vi "UpdateLaserAOTFSettings.vi"(0 "3.LaserChannel ON/OFF":bool, 1 "4.LaserChannel ON/OFF":bool, 2 "On/OFF  Power 2":bool, 3 "6.LaserChannel ON/OFF":bool, 4 "7.LaserChannel ON/OFF":bool, 5 "8.LaserChannel ON/OFF":bool, 6 "1.Laser Channel Power / [%]":i16 min=0 max=100 step=1, 7 "2.Laser Channel Power / [%]":i16 min=0 max=100 step=1, 8 "2.LaserChannel ON/OFF":bool, 9 "3.Laser Channel Power / [%]":i16 min=0 max=100 step=1, 10 "On/OFF  Power":bool, 11 "4.Laser Channel Power / [%]":i16 min=0 max=100 step=1, 13 "5.Laser Channel Power / [%]":i16 min=0 max=100 step=1, 14 "error in":errorcluster, 15 "6.Laser Channel Power / [%]":i16 min=0 max=100 step=1, 17 "7.Laser Channel Power / [%]":i16 min=0 max=100 step=1, 19 "8.Laser Channel Power / [%]":i16 min=0 max=100 step=1, 20 "1.Laser Channel Wavelength 8":i32, 21 "1.Laser Channel Wavelength 7":i32, 22 "1.Laser Channel Wavelength 6":i32, 23 "Wavelength 2":i32, 24 "1.Laser Channel Wavelength 4":i32, 25 "1.Laser Channel Wavelength 3":i32, 26 "1.Laser Channel Wavelength 2":i32, 27 "Wavelength":i32) -> (18 "error out":errorcluster)   [LabVIEW 2013]
uses:
  Variables/AOTF_NonLinearLinesOnOff.vi
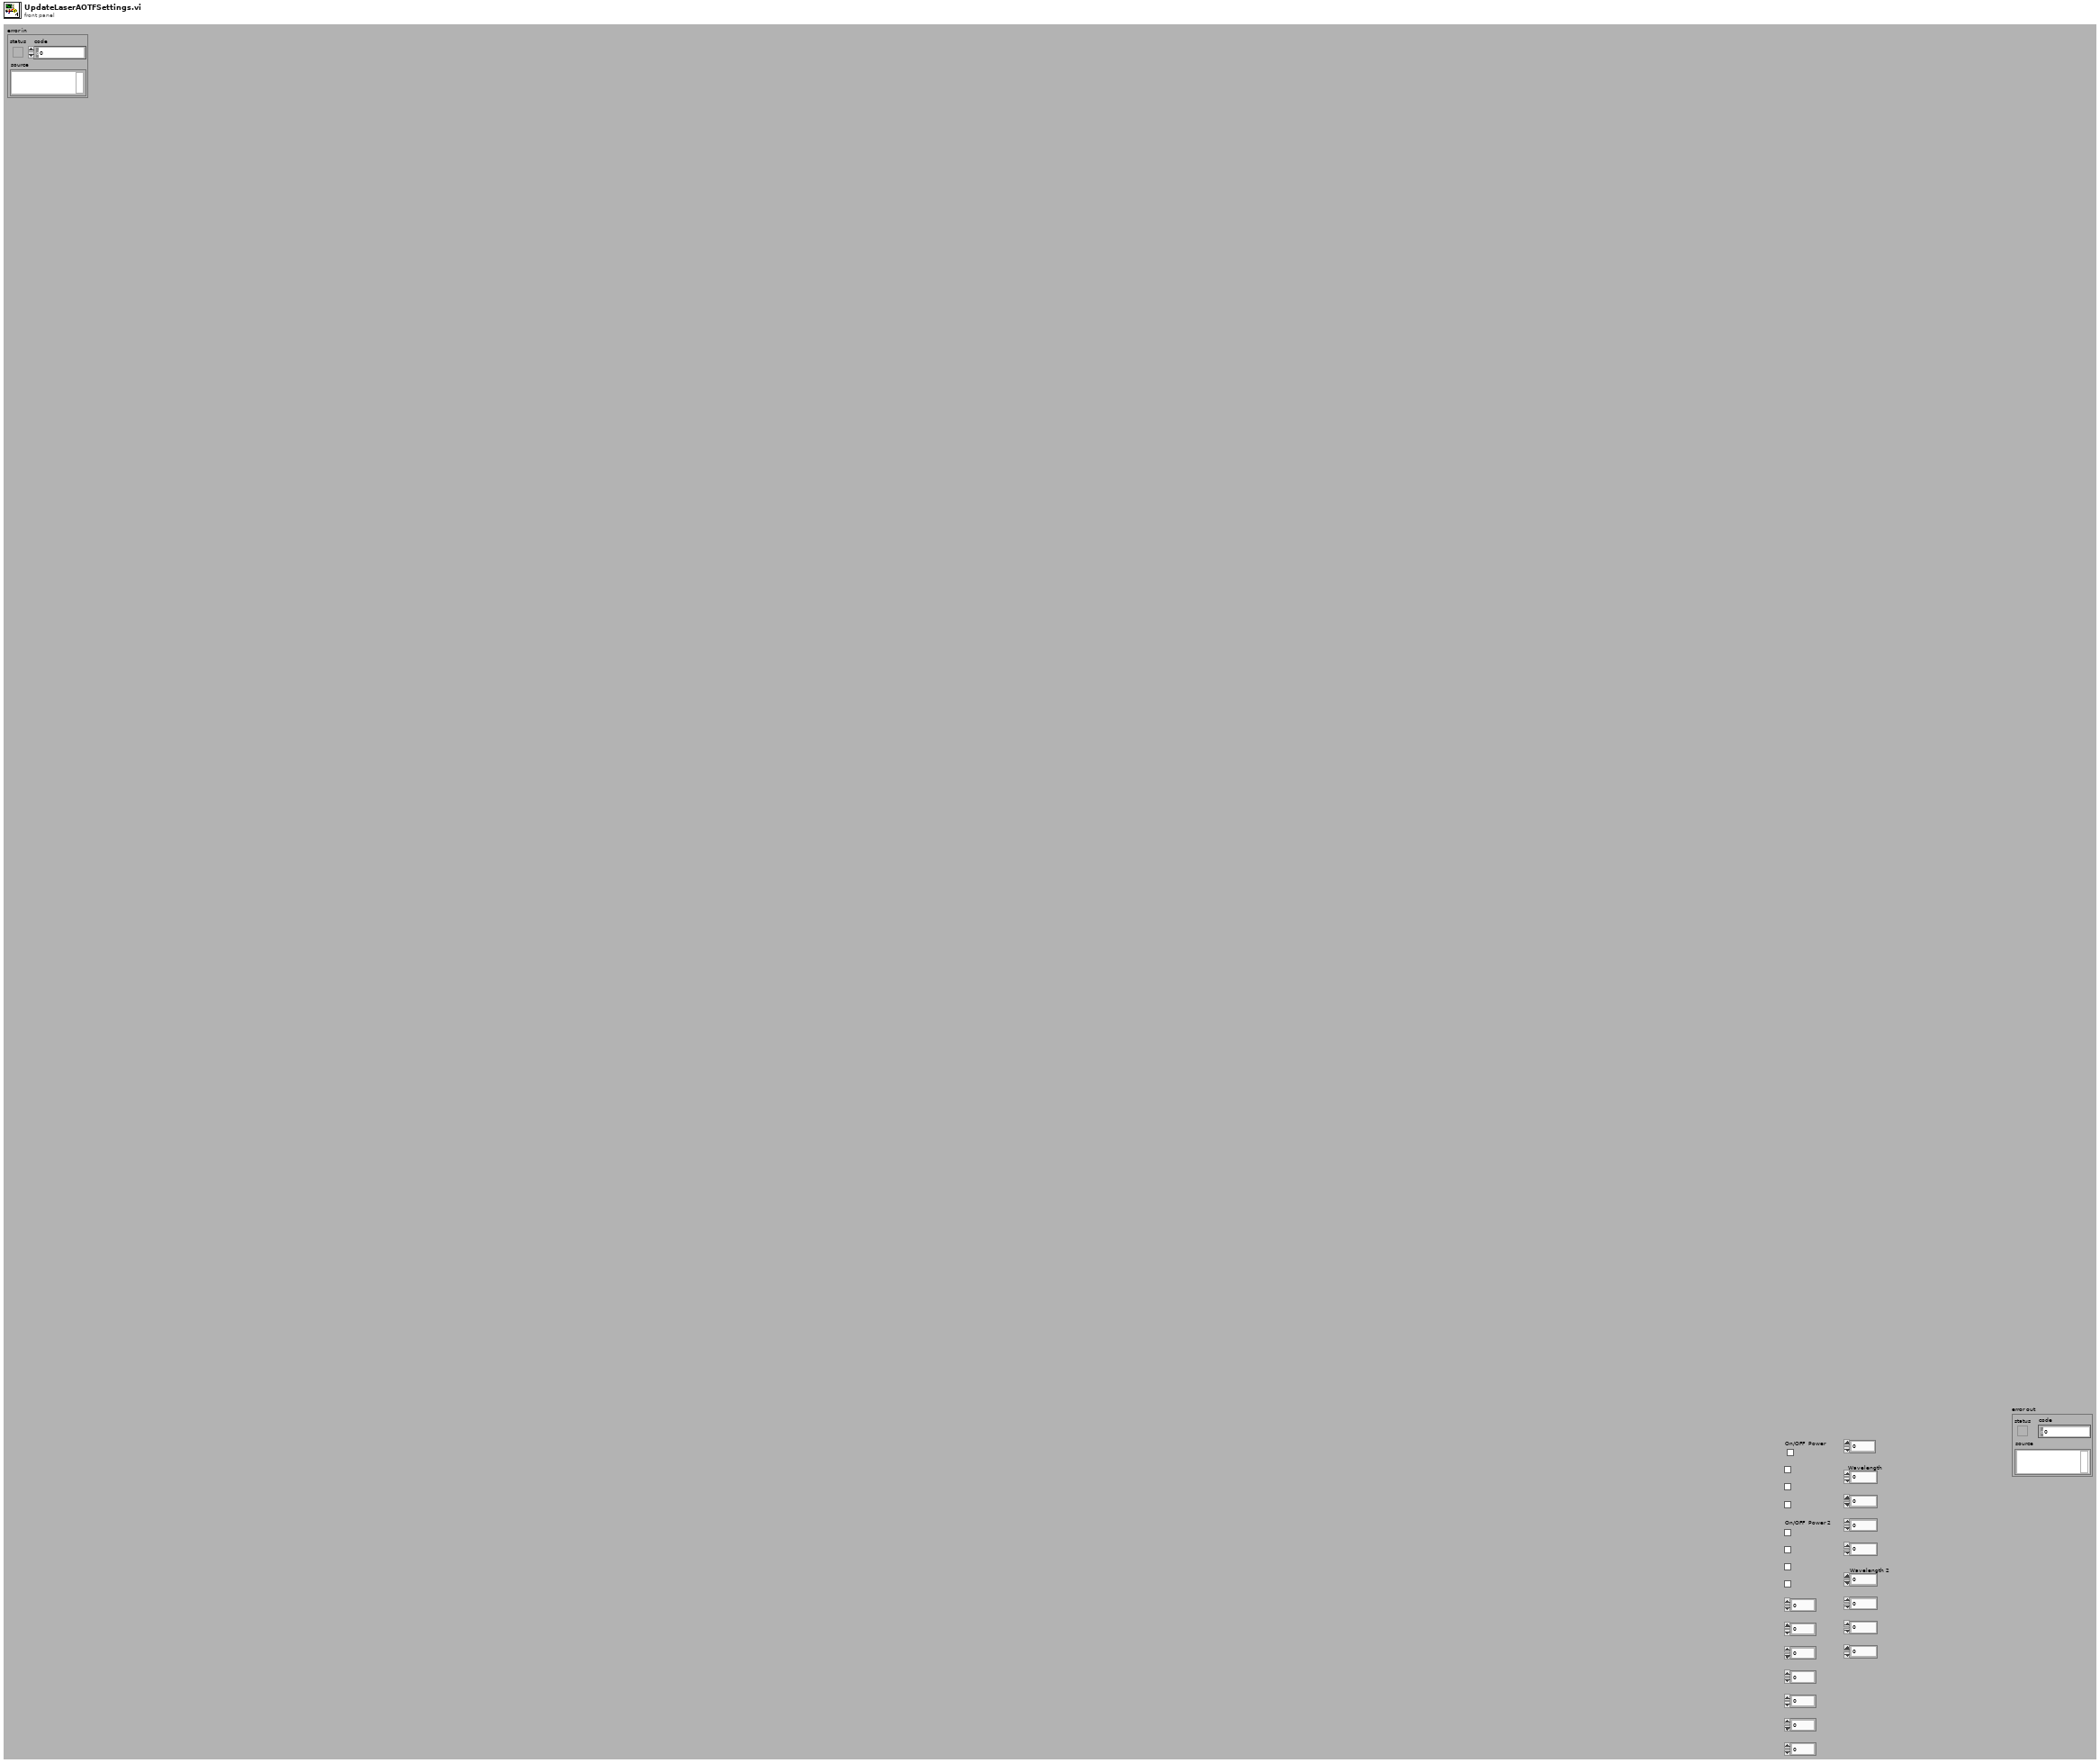
[diagram p1: front panel]
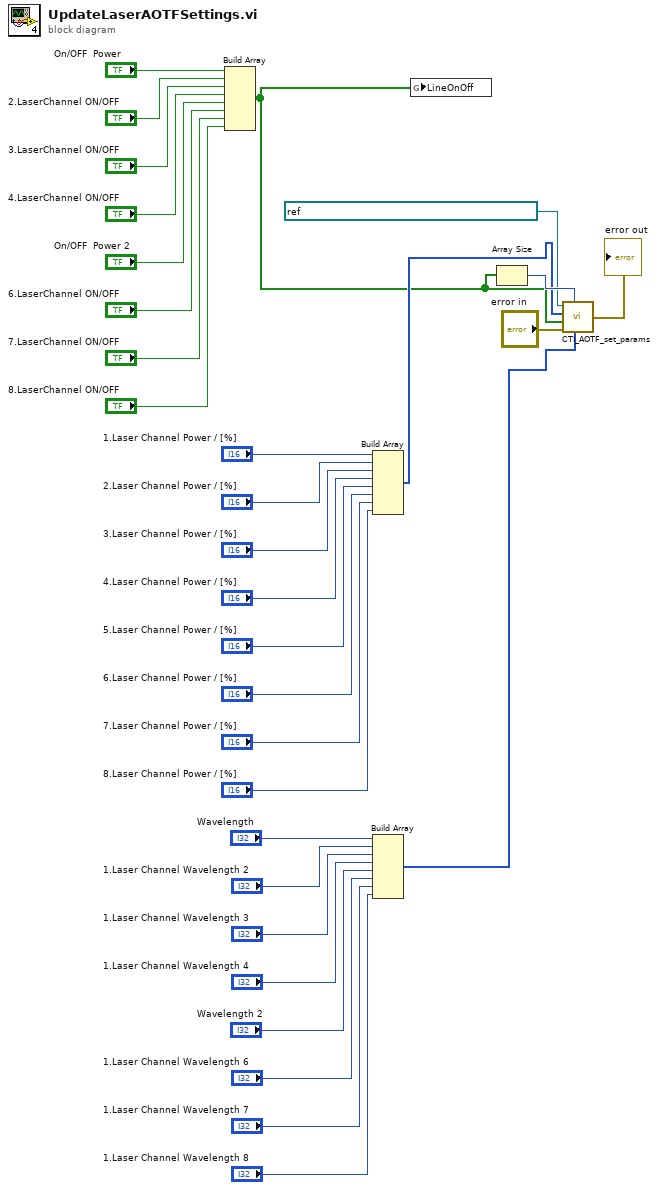
[diagram p0: block diagram]
diagram:
  n1 = Build Array("On/OFF  Power", "2.LaserChannel ON/OFF", "3.LaserChannel ON/OFF", "4.LaserChannel ON/OFF", "On/OFF  Power 2", "6.LaserChannel ON/OFF", "7.LaserChannel ON/OFF", "8.LaserChannel ON/OFF") -> (w1:bool[])
  n2 = Build Array("1.Laser Channel Power / [%]", "2.Laser Channel Power / [%]", "3.Laser Channel Power / [%]", "4.Laser Channel Power / [%]", "5.Laser Channel Power / [%]", "6.Laser Channel Power / [%]", "7.Laser Channel Power / [%]", "8.Laser Channel Power / [%]") -> (w4:i16[])
  n3 = Build Array("Wavelength", "1.Laser Channel Wavelength 2", "1.Laser Channel Wavelength 3", "1.Laser Channel Wavelength 4", "Wavelength 2", "1.Laser Channel Wavelength 6", "1.Laser Channel Wavelength 7", "1.Laser Channel Wavelength 8") -> (w3:i32[])
  n4 = global write "AOTF_NonLinearLinesOnOff.vi" "LineOnOff"(w1) -> ()
  n5 = Array Size(array=w1) -> (size(s)=w7:i32)
  n6 = call "CTI_AOTF_set_params.vi"("frequency"=w3, "Numeric"=w7, "error IO"="error in", "Array"=w1, "amplitude"=w4, "CTI AOTF-Controller"=refnum<visa-resource-name> "USB0::0x16C7::0x0001::NI-VISA-20001::RAW" ("VISA resource name 2")) -> ("error out"=→"error out":errorcluster)
